vi "usrp get normalized rx gain.vi"(8 "error in (no error)":errorcluster, 9 "gain_out":dbl, 10 "chan":u64, 11 "h":u64) -> (0 "error out":errorcluster, 1 "gain_out out":dbl, 3 "function return":u32(ring))   [LabVIEW 2023, in "uhd.lvlib"]
doc: "UHD_API uhd_error uhd_usrp_get_normalized_rx_gain(\n uhd_usrp_handle h, size_t chan, double* gain_out);"
uses:
  <userlib>/uhd/uhd.lvlib
  <userlib>/uhd/uhd.dll
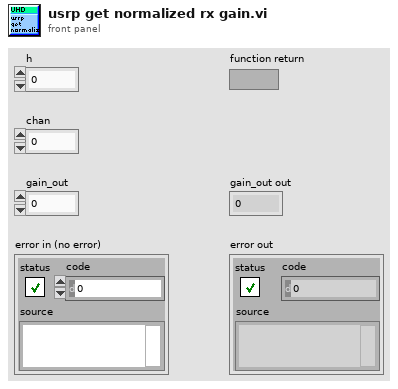
[diagram p1: front panel]
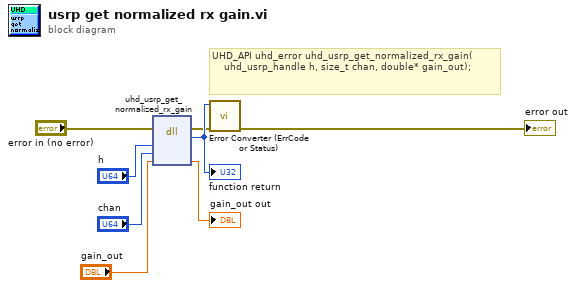
[diagram p0: block diagram]
diagram:
  # "UHD_API uhd_error uhd_usrp_get_normalized_rx_gain(\n    uhd_usrp_handle h, size_t chan, double* gain_out);"
  n1 = dll-call lib="C:/Program Files/National Instruments/LabVIEW 2023/user.lib/uhd/uhd.*" fn="uhd_usrp_get_normalized_rx_gain"(error in="error in (no error)", "h"="h", "chan"="chan", "gain_out"="gain_out") -> (error out=w2:errorcluster, w8:u32, "gain_out"=→"gain_out out":dbl)  [unwired: 4 in, 1 out]
  "function return" <- w8
  n2 = call <userlib>:"Error Converter (ErrCode or Status).vi"("error in (no error)"=w2, "error code"=w8) -> ("error out"=→"error out":errorcluster)  [unwired: 9 in]
